vi "Construct_Optimal_Subtrack_(101)-1.vi"(6 "[IN] Indexes for Jumps":i32[](array[numeric]), 8 "error IN":errorcluster, 9 "[IN] Index of recon\nstructed tracks":i32, 10 "[IN] Clusters for Re\nconstructed Tracks":T1, 11 "[IN] Still connected\ntracks in group":T2) -> (0 "error OUT":errorcluster, 2 "[OUT] Clusters for Re\nconstructed Tracks":T1)   [LabVIEW 2013]
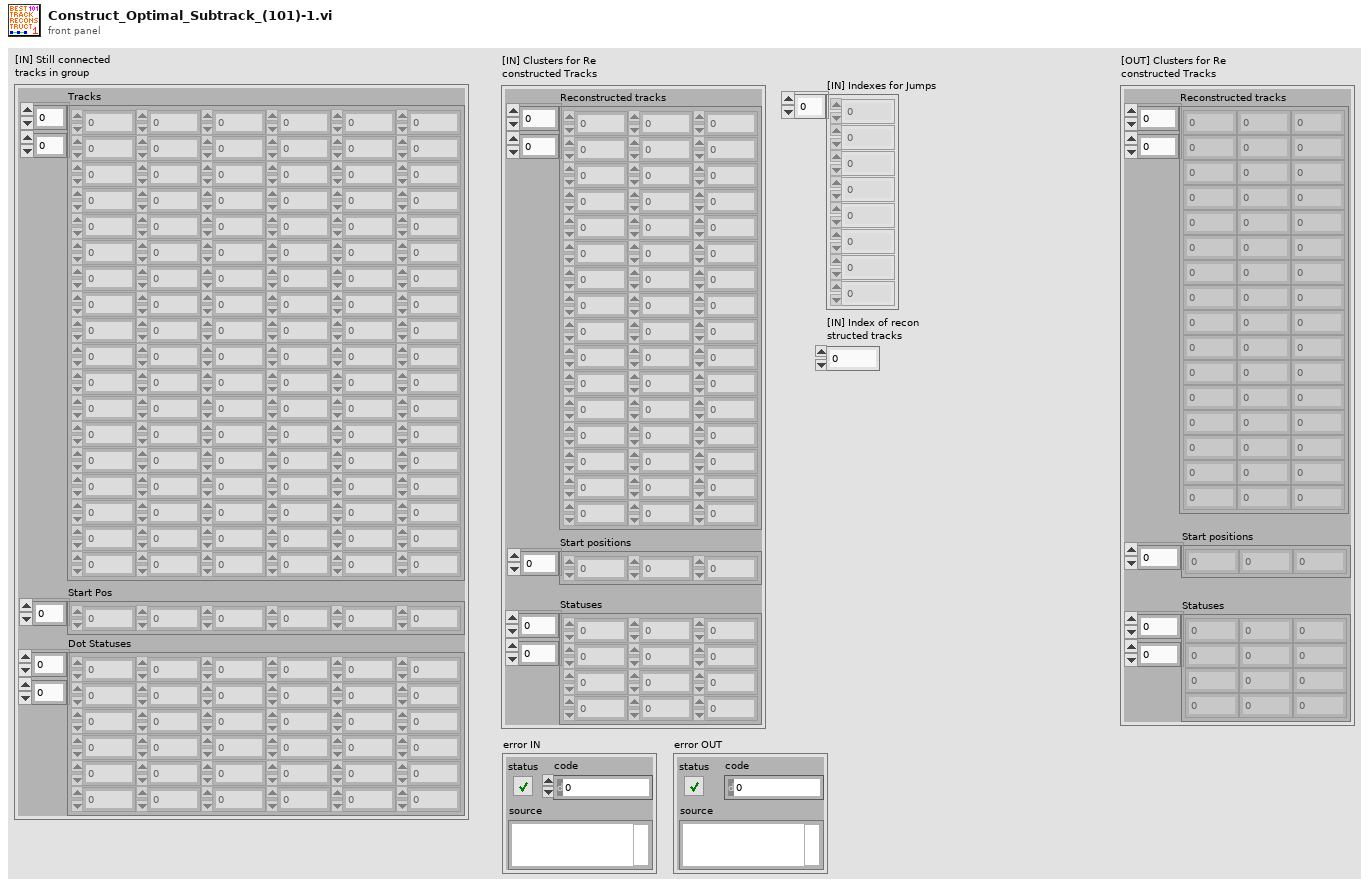
[diagram p1: front panel]
types:
  T1 = cluster{"Reconstructed tracks":dbl[][], "Start positions":i32[], "Statuses":i16[][]}
  T2 = cluster{"Tracks":dbl[][], "Start Pos":i32[], "Dot Statuses":i16[][]}
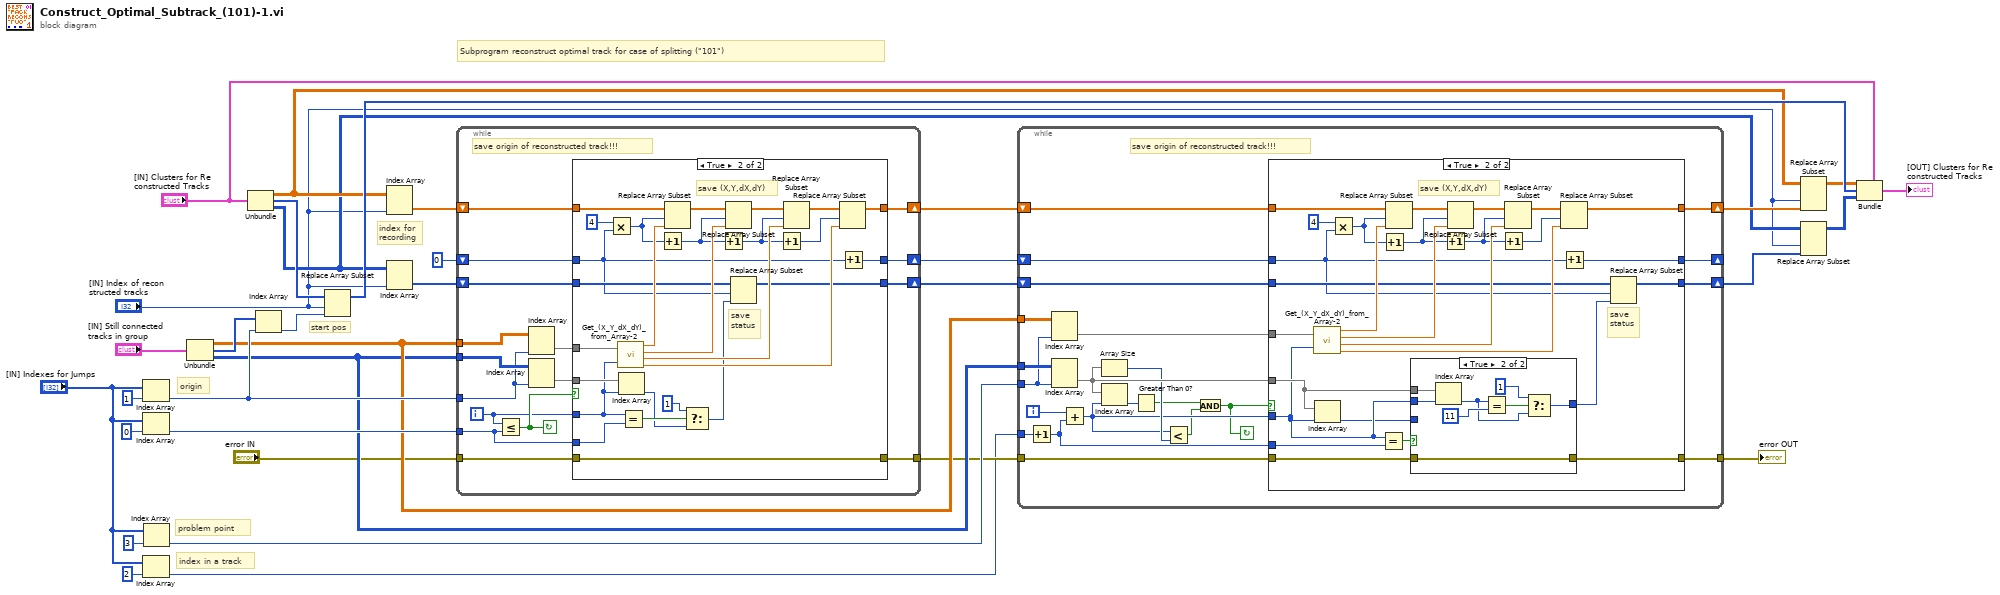
[diagram p0: block diagram]
diagram:
  # "index in a track"
  # "problem point"
  # "origin"
  # "Subprogram reconstruct optimal track for case of splitting (\"101\")"
  # "index for\nrecording"
  # "start pos"
  n1 = Index Array(array="[IN] Indexes for Jumps", index=1) -> (element=w25:i32)
  n2 = Index Array(array="[IN] Indexes for Jumps", index=0) -> (element=w28:i32)
  n3 = Index Array(array="[IN] Indexes for Jumps", index=2) -> (element=w1:i32)
  n4 = Index Array(array="[IN] Indexes for Jumps", index=3) -> (element=w15:i32)
  n5 = Unbundle("[IN] Still connected\ntracks in group") -> ("Tracks"=w17:dbl[][], "Start Pos"=w26:i32[], "Dot Statuses"=w16:i16[][])
  n6 = Unbundle("[IN] Clusters for Re\nconstructed Tracks") -> ("Reconstructed tracks"=w12:dbl[][], "Start positions"=w27:i32[], "Statuses"=w9:i16[][])
  n7 = Index Array(array=w26, index=w25) -> (element=w24:i32)
  n8 = Replace Array Subset(array=w27, new element=w24, index="[IN] Index of recon\nstructed tracks") -> (w13:i32[])
  n9 = Index Array(array=w12, index (col)="[IN] Index of recon\nstructed tracks") -> (element=w23:dbl[])  [unwired: 1 in]
  n10 = Index Array(array=w9, index (col)="[IN] Index of recon\nstructed tracks") -> (element=w22:i16[])  [unwired: 1 in]
  n11 = while {
    tunnel: w28 -> [w35]
    tunnel: w17 -> [w50]
    tunnel: w16 -> [w49]
    tunnel: w25 -> [w48]
    shift-right: [w40] -> w20
    shift-left: w23 -> [w46]
    shift-right: [w38] -> w18
    shift-left: w22 -> [w42]
    shift-right: [w39] -> w19
    shift-left: 0 -> [w41]
    tunnel: "error IN" -> [w37]
    tunnel: [w36] -> w3
    i -> [w43]
    stop <- w47 continue-if-true
    # "save origin of reconstructed track!!!"
    n12 = Less Or Equal?(x=w43, y=w35) -> (x <= y?=w47:bool)
    n13 = Index Array(array=w50, index (col)=w48) -> (element=w45:dbl[])  [unwired: 1 in]
    n14 = Index Array(array=w49, index (col)=w48) -> (element=w44:i16[])  [unwired: 1 in]
    n15 = case shown="True" w47 {
      tunnel: w46 -> [w54 w79]
      tunnel: w45 -> [_ w81]
      tunnel: w44 -> [_ w80]
      tunnel: w43 -> [_ w58]
      tunnel: w42 -> [w52 w66]
      tunnel: [w52 w65] -> w38
      tunnel: [w54 w64] -> w40
      tunnel: w41 -> [w53 w63]
      tunnel: [w53 w62] -> w39
      tunnel: w37 -> [w51 w61]
      tunnel: [w51 w61] -> w36
      tunnel: w35 -> [_ w57]
      frame False {
      }
      frame True {
        # "save (X,Y,dX,dY)"
        # "save\nstatus"
        n16 = Multiply(x=4, y=w63) -> (x*y=w75:i32)
        n17 = call "Get_(X_Y_dX_dY)_from_Array-2.vi"("(X,Y,dX,dY)"=w81, "Index of Displacement"=w58) -> ("X"=w77:dbl, "Y"=w74:dbl, "dX"=w71:dbl, "dY"=w67:dbl)
        n18 = Index Array(array=w80, index=w58) -> (element=w55:i16)
        n19 = Equal?(x=w58, y=w57) -> (x = y?=w59:bool)
        n20 = Increment(x=w75) -> (x+1=w72:i32)
        n21 = Replace Array Subset(array=w79, new element=w77, index=w75) -> (w76:dbl[])
        n22 = Select(t=i16 1, s=w59, f=w55) -> (s? t:f=w56:i16)
        n23 = Increment(x=w72) -> (x+1=w70:i32)
        n24 = Replace Array Subset(array=w76, new element=w74, index=w72) -> (w73:dbl[])
        n25 = Replace Array Subset(array=w66, new element=w56, index=w63) -> (w65:i16[])
        n26 = Increment(x=w70) -> (x+1=w69:i32)
        n27 = Replace Array Subset(array=w73, new element=w71, index=w70) -> (w68:dbl[])
        n28 = Replace Array Subset(array=w68, new element=w67, index=w69) -> (w64:dbl[])
        n29 = Increment(x=w63) -> (x+1=w62:i32)
      }
    }
  }
  n30 = while {
    tunnel: w17 -> [w103]
    tunnel: w16 -> [w102]
    tunnel: w15 -> [w101]
    shift-right: [w96] -> w11
    shift-left: w20 -> [w100]
    shift-right: [w94] -> w8
    shift-left: w18 -> [w98]
    shift-right: [w95] -> _
    shift-left: w19 -> [w97]
    tunnel: w1 -> [w83]
    tunnel: w3 -> [w85]
    tunnel: [w84] -> w2
    i -> [w93]
    stop <- w86 continue-if-true
    # "save origin of reconstructed track!!!"
    n31 = Increment(x=w83) -> (x+1=w82:i32)
    n32 = Index Array(array=w103, index (col)=w101) -> (element=w99:dbl[])  [unwired: 1 in]
    n33 = Index Array(array=w102, index (col)=w101) -> (element=w92:i16[])  [unwired: 1 in]
    n34 = Add(x=w93, y=w82) -> (x+y=w89:i32)
    n35 = Array Size(array=w92) -> (size(s)=w90:i32)
    n36 = Index Array(array=w92, index=w89) -> (element=w91:i16)
    n37 = Greater Than 0?(x=w91) -> (x > 0?=w88:bool)
    n38 = Less?(x=w89, y=w90) -> (x < y?=w87:bool)
    n39 = And(x=w88, y=w87) -> (x .and. y?=w86:bool)
    n40 = case shown="True" w86 {
      tunnel: w100 -> [w107 w133]
      tunnel: w99 -> [_ w134]
      tunnel: w92 -> [_ w114]
      tunnel: w89 -> [_ w110]
      tunnel: w98 -> [w105 w120]
      tunnel: [w105 w119] -> w94
      tunnel: [w107 w118] -> w96
      tunnel: w97 -> [w106 w117]
      tunnel: [w106 w116] -> w95
      tunnel: w85 -> [w104 w112]
      tunnel: [w104 w111] -> w84
      tunnel: w82 -> [_ w108]
      frame False {
      }
      frame True {
        # "save (X,Y,dX,dY)"
        # "save\nstatus"
        n41 = call "Get_(X_Y_dX_dY)_from_Array-2.vi"("(X,Y,dX,dY)"=w134, "Index of Displacement"=w110) -> ("X"=w131:dbl, "Y"=w128:dbl, "dX"=w125:dbl, "dY"=w121:dbl)
        n42 = Index Array(array=w114, index=w110) -> (element=w109:i16)
        n43 = Multiply(x=4, y=w117) -> (x*y=w129:i32)
        n44 = Equal?(x=w110, y=w108) -> (x = y?=w115:bool)
        n45 = Increment(x=w129) -> (x+1=w126:i32)
        n46 = Replace Array Subset(array=w133, new element=w131, index=w129) -> (w130:dbl[])
        n47 = case shown="True" w115 {
          tunnel: w109 -> [w136 _]
          tunnel: w110 -> [_ w144]
          tunnel: w114 -> [_ w143]
          tunnel: [w136 w137] -> w113
          tunnel: w112 -> [w135 w139]
          tunnel: [w135 w139] -> w111
          frame False {
          }
          frame True {
            n48 = Index Array(array=w143, index=w144) -> (element=w138:i16)
            n49 = Equal?(x=w138, y=i16 11) -> (x = y?=w141:bool)
            n50 = Select(t=i16 1, s=w141, f=w138) -> (s? t:f=w137:i16)
          }
        }
        n51 = Increment(x=w126) -> (x+1=w124:i32)
        n52 = Replace Array Subset(array=w130, new element=w128, index=w126) -> (w127:dbl[])
        n53 = Increment(x=w124) -> (x+1=w123:i32)
        n54 = Replace Array Subset(array=w127, new element=w125, index=w124) -> (w122:dbl[])
        n55 = Replace Array Subset(array=w122, new element=w121, index=w123) -> (w118:dbl[])
        n56 = Increment(x=w117) -> (x+1=w116:i32)
        n57 = Replace Array Subset(array=w120, new element=w113, index=w117) -> (w119:i16[])
      }
    }
  }
  "error OUT" <- w2
  n58 = Replace Array Subset(array=w12, new element=w11, index (col)="[IN] Index of recon\nstructed tracks") -> (w10:dbl[][])  [unwired: 1 in]
  n59 = Replace Array Subset(array=w9, new element=w8, index (col)="[IN] Index of recon\nstructed tracks") -> (w6:i16[][])  [unwired: 1 in]
  n60 = Bundle(cluster="[IN] Clusters for Re\nconstructed Tracks", "Reconstructed tracks"=w10, "Start positions"=w13, "Statuses"=w6) -> (→"[OUT] Clusters for Re\nconstructed Tracks":T1)
